vi "Remove Constant Strings.vi"(0 "Function String":string, 11 "error in (no error)":errorcluster) -> (4 "Replace Sub Function with variable":string, 6 "Constant String":string[](array[string]), 8 "Variables":string[](array[string]), 15 "error out":errorcluster)   [LabVIEW 2019]
panel:
  # "function_name(a=1,\"0,1\",a++)"
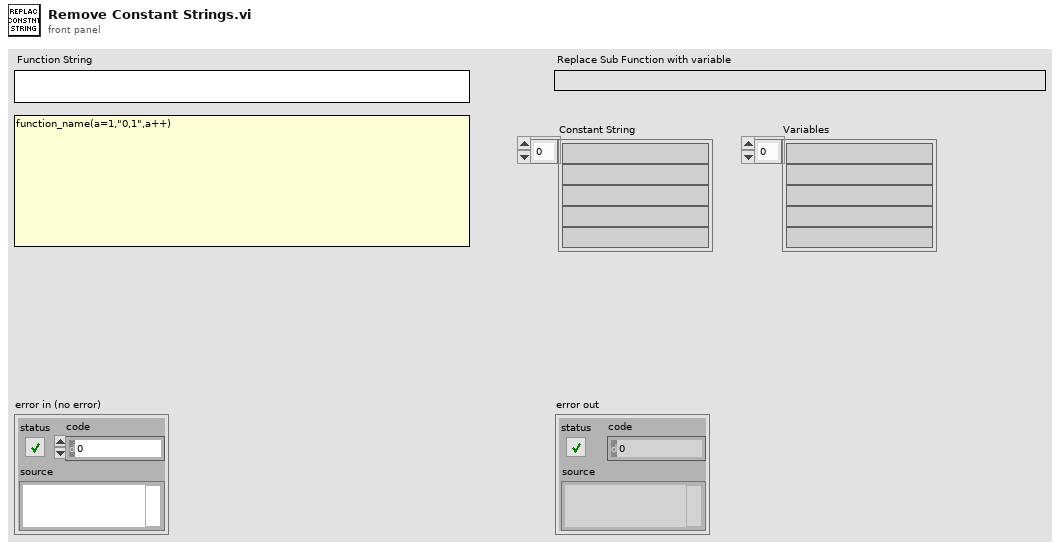
[diagram p1: front panel]
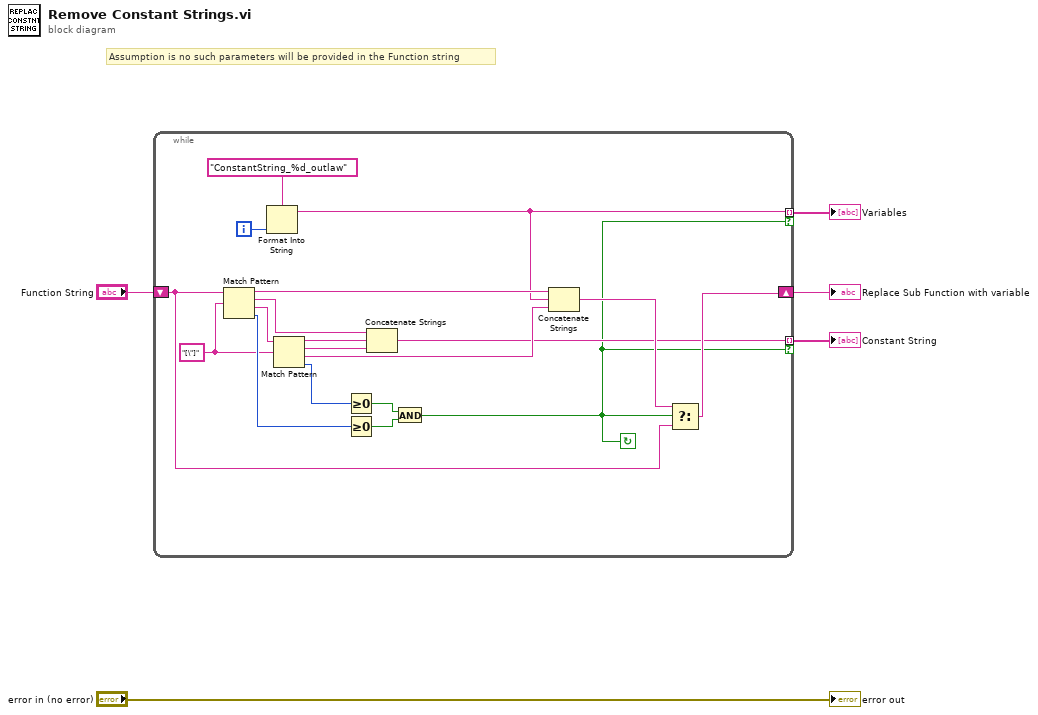
[diagram p0: block diagram]
diagram:
  # "Assumption is no such parameters will be provided in the Function string"
  n1 = while {
    shift-right: [w12] -> w3
    shift-left: "Function String" -> [w11]
    tunnel: [w10] -> w2 mode=indexing if=w6
    tunnel: [w7] -> w1 mode=indexing if=w6
    i -> [w19]
    stop <- w6 continue-if-true
    w22 = "[\"]" ("regular expression")
    n2 = Match Pattern(string=w11, regular expression=w22) -> (before substring=w15:string, match substring=w8:string, after substring=w23:string, offset past match=w24:i32)  [unwired: 1 in]
    n3 = Format Into String(format string="ConstantString_%d_outlaw", w19) -> (resulting string=w7:string)  [unwired: 2 in, 1 out]
    n4 = Match Pattern(string=w23, regular expression=w22) -> (before substring=w21:string, match substring=w9:string, after substring=w14:string, offset past match=w18:i32)  [unwired: 1 in]
    n5 = Greater Or Equal To 0?(x=w18) -> (x >= 0?=w17:bool)
    n6 = Greater Or Equal To 0?(x=w24) -> (x >= 0?=w16:bool)
    n7 = Concatenate Strings(w8, w21, w9) -> (w10:string)
    n8 = And(x=w17, y=w16) -> (x .and. y?=w6:bool)
    n9 = Concatenate Strings(w15, w7, w14) -> (w13:string)
    n10 = Select(t=w13, s=w6, f=w11) -> (s? t:f=w12:string)
  }
  "Replace Sub Function with variable" <- w3
  "Constant String" <- w2
  "Variables" <- w1
  "error out" <- "error in (no error)"
